vi "Simulated LIDAR (Faster).vi"(8 "error in (no error)":errorcluster, 9 "End Point (120°)":dbl=120.0, 10 "Start Point (-120°)":dbl=-120.0) -> (0 "error out":errorcluster, 1 "Direction":dbl[](array[numeric]), 2 "Magnitude":dbl[](array[numeric]))   [LabVIEW 2011]
doc: "This VI takes three parameters (start point, end point, cluster count) and returns two arrays which describe the magnitude and angle at which the data was acquired. \n\nThe reference for the angles (in the Direction array) is the center of the device which is 0° with positive angles to the left of center and negative angles to the right.\n\nThe URG-04LX can take measurements in the range of -120° to 120° and has an \"operating range\" of -135° to 135°. \n\nCluster Count refers to the number of measurements which are clustered together. \n<b>Ex:</b>If the cluster count is 3 then the smallest of three measurements is returned.\n\nThe Magnitude array is associated with the Direction array. \n<b>Ex:</b> If the information for the first measurement is desired, then the 0th index of each array is accessed and returns the magnitude and direction of the first measurement.\n\nIf checksums are being used and the checksum fails, the data returned in the magnitude array will default to -1."
uses:
  2D Point.ctl
  <vilib>/Analysis/coordinate.llb/Wrap Angle (scalar).vi
  <vilib>/Analysis/coordinate.llb/2D Cartesian Coordinate Rotation (Scalar).vi
  <vilib>/Utility/AngleManip/Radians to Degrees (Scalar DBL).vi
  <vilib>/Utility/AngleManip/Degrees to Radians (Scalar DBL).vi
  <vilib>/Analysis/NI_AALPro.lvlib
  <vilib>/Analysis/NI_AALBase.lvlib
  <vilib>/Utility/AngleManip/NI_AngleManipulation.lvlib
  <vilib>/Analysis/NI_AAL_Angle.lvlib
panel:
  in  "Add noise?":bool=TRUE
  in  "noise (standard deviation)":dbl=30.0
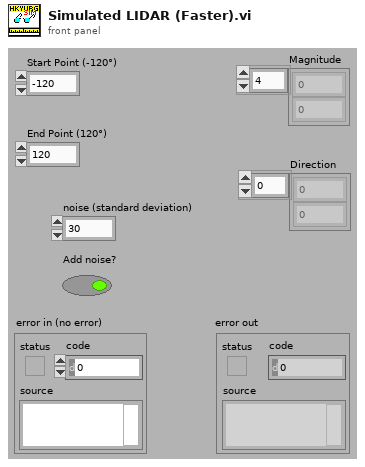
[diagram p1: front panel]
types:
  T1 = typedef "2D Point.ctl" = cluster{"X":dbl, "Y":dbl}
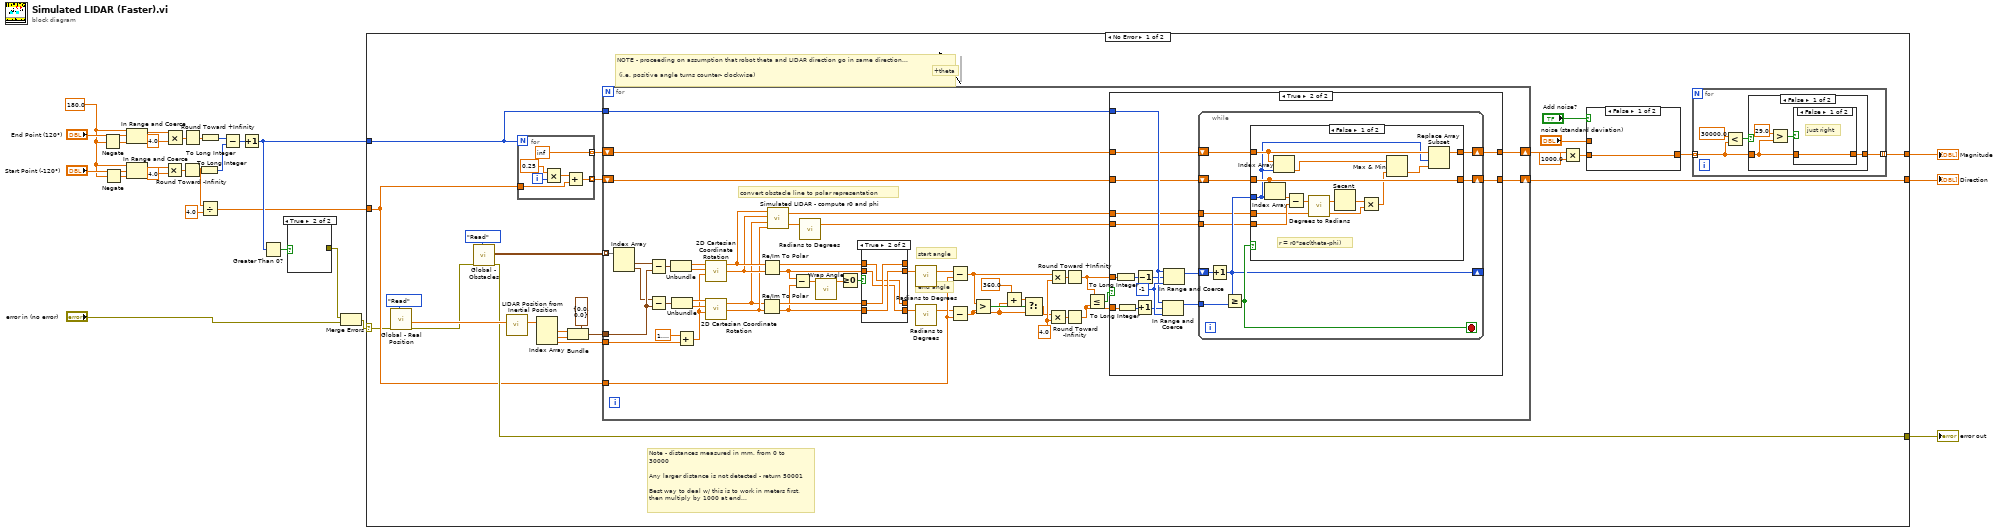
[diagram p0: block diagram]
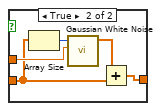
[diagram p2: hidden frame]
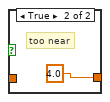
[diagram p3: hidden frame]
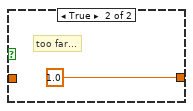
[diagram p4: hidden frame]
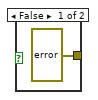
[diagram p9: hidden frame]
diagram:
  w20 = 180.0 ("upper limit")
  n1 = Negate(x=w20) -> (-x=w22:dbl)
  n2 = Negate(x=w20) -> (-x=w23:dbl)
  n3 = In Range and Coerce(upper limit=w20, x="End Point (120°)", lower limit=w22) -> (coerced(x)=w18:dbl)  [unwired: 1 out]
  n4 = In Range and Coerce(upper limit=w20, x="Start Point (-120°)", lower limit=w23) -> (coerced(x)=w19:dbl)  [unwired: 1 out]
  n5 = Multiply(x=w19, y=4.0) -> (x*y=w6:dbl)
  n6 = Multiply(x=w18, y=4.0) -> (x*y=w25:dbl)
  n7 = Round Toward -Infinity(1:w6) -> (0:w4:dbl)
  n8 = Round Toward +Infinity(x=w25) -> (ceil(x): smallest int >= x=w17:dbl)
  n9 = To Long Integer(number=w4) -> (32bit integer=w16:i32)
  n10 = To Long Integer(number=w17) -> (32bit integer=w15:i32)
  n11 = Divide(x=w4, y=4.0) -> (x/y=w3:dbl)
  n12 = Subtract(x=w15, y=w16) -> (x-y=w14:i32)
  n13 = Increment(x=w14) -> (x+1=w11:i32)
  n14 = Greater Than 0?(x=w11) -> (x > 0?=w9:bool)
  n15 = case shown="True" w9 {
    tunnel: [errorcluster {"status"=TRUE, "code"=1, "source"="Simulated LIDAR: Check Start and End Points"} ("t") _] -> w8
    frame False {
    }
    frame True {
    }
  }
  n16 = Merge Errors(w8, "error in (no error)") -> (w7:errorcluster)
  n17 = case shown="No Error" w7 {
    selector: w7 -> [w28 _]
    tunnel: [w44 _] -> w12
    tunnel: w11 -> [w37 _]
    tunnel: w3 -> [w38 _]
    tunnel: [w36 _] -> w2
    tunnel: [w34 _] -> w1
    frame No Error {
      # "NOTE - proceeding on assumption that robot theta and LIDAR direction go in same direction...\n\n (i.e. positive angle turns counter- clockwise)"
      # "+theta"
      # "Note - distances measured in mm, from 0 to 30000\n\nAny larger distance is not detected - return 50001\n\nBest way to deal w/ this is to work in meters first, then multiply by 1000 at end..."
      n18 = call "Global - Real Position.vi"("mode"=enum16{"Initialize", "Read", "Write"}."Read" ("Mode"), "error in (no error)"=w28) -> ("error out"=w46:errorcluster, "real x, y, theta out"=w48:dbl[])  [unwired: 7 in, 1 out]
      n19 = call "Global - Obstacles.vi"("mode"=enum16{"Initialize", "Read", "Write"}."Read" ("Mode"), "error in (no error)"=w46) -> ("error out"=w44:errorcluster, "obstacles out"=w43:cluster{dbl, dbl}[][])  [unwired: 7 in, 1 out]
      n20 = call "LIDAR Position from Inertial Position.vi"("CM X, Y, Theta"=w48) -> ("LIDAR X, Y, Theta"=w47:dbl[])  [unwired: 1 in, 9 out]
      n21 = for {
        N: w37 -> [_]
        tunnel: [inf] -> w39 mode=indexing
        tunnel: w38 -> [w71]
        tunnel: [w70] -> w40 mode=indexing
        i -> [w74]
        n22 = Multiply(x=0.25, y=w74) -> (x*y=w73:dbl)
        n23 = Add(x=w73, y=w71) -> (x+y=w70:dbl)
      }
      n24 = Index Array(array=w47) -> (element #1=w51:dbl, element #2=w50:dbl, element #3=w41:dbl)  [unwired: 3 in]
      n25 = Bundle(cluster=T1 {"X"=0.0, "Y"=0.0} ("2D Point"), "X"=w51, "Y"=w50) -> (w42:T1)
      n26 = for {
        tunnel: w43 -> [w124] mode=indexing
        tunnel: w42 -> [w123]
        tunnel: w41 -> [w86]
        shift-right: [w88] -> w36
        shift-left: w40 -> [w89]
        shift-right: [w90] -> w33
        shift-left: w39 -> [w91]
        tunnel: w38 -> [w105]
        tunnel: w37 -> [w101]
        w104 = 4.0 ("y")
        # "convert obstacle line to polar representation"
        # "end angle"
        # "start angle"
        n27 = Index Array(array=w124) -> (element #1=w122:cluster{dbl, dbl}, element #2=w121:cluster{dbl, dbl})  [unwired: 2 in]
        n28 = Subtract(x=w122, y=w123) -> (x-y=w120:T1)
        n29 = Subtract(x=w121, y=w123) -> (x-y=w119:T1)
        n30 = Unbundle(w120) -> ("X"=w118:dbl, "Y"=w117:dbl)
        n31 = Unbundle(w119) -> ("X"=w116:dbl, "Y"=w115:dbl)
        n32 = Add(x=1.5707963267948966, y=w86) -> (x+y=w85:dbl)
        n33 = call-poly <vilib>:"2D Cartesian Coordinate Rotation.vi"("theta"=w85, "y"=w117, "x"=w118) -> ("y out"=w108:dbl, "x out"=w109:dbl)  [unwired: 6 in, 1 out]
        n34 = call-poly <vilib>:"2D Cartesian Coordinate Rotation.vi"("theta"=w85, "y"=w115, "x"=w116) -> ("y out"=w107:dbl, "x out"=w106:dbl)  [unwired: 6 in, 1 out]
        n35 = Re/Im To Polar(2:w107, 3:w106) -> (0:w110:dbl, 1:w111:dbl)
        n36 = Re/Im To Polar(2:w108, 3:w109) -> (0:w112:dbl, 1:w113:dbl)
        n37 = call "Simulated LIDAR - compute r0 and phi.vi"("y2"=w107, "x2"=w106, "y1"=w108, "x1"=w109) -> ("phi"=w83:dbl, "r0"=w87:dbl)
        n38 = Subtract(x=w112, y=w110) -> (x-y=w77:dbl)
        n39 = call-poly <vilib>:"Radians to Degrees.vi"("angle (rad)"=w83) -> ("angle (deg)"=w82:dbl)  [unwired: 2 in]
        n40 = call-poly <vilib>:"Wrap Angle.vi"("angle in"=w77) -> ("angle out"=w76:dbl)  [unwired: 9 in, 1 out]
        n41 = Greater Or Equal To 0?(x=w76) -> (x >= 0?=w114:bool)
        n42 = case shown="True" w114 {
          tunnel: w113 -> [w171 w173]
          tunnel: w112 -> [w170 w172]
          tunnel: w111 -> [w169 w175]
          tunnel: w110 -> [w168 w174]
          tunnel: [w171 w175] -> _
          tunnel: [w170 w174] -> w79
          tunnel: [w169 w173] -> _
          tunnel: [w168 w172] -> w81
          frame False {
          }
          frame True {
          }
        }
        n43 = call-poly <vilib>:"Radians to Degrees.vi"("angle (rad)"=w79) -> ("angle (deg)"=w78:dbl)  [unwired: 2 in]
        n44 = call-poly <vilib>:"Radians to Degrees.vi"("angle (rad)"=w81) -> ("angle (deg)"=w80:dbl)  [unwired: 2 in]
        n45 = Subtract(x=w78, y=w105) -> (x-y=w100:dbl)
        n46 = Subtract(x=w80, y=w105) -> (x-y=w96:dbl)
        n47 = Greater?(x=w100, y=w96) -> (0:w97:bool)
        n48 = Add(x=360.0, y=w96) -> (x+y=w99:dbl)
        n49 = Select(t=w99, s=w97, f=w96) -> (s? t:f=w95:dbl)
        n50 = Multiply(x=w95, y=w104) -> (x*y=w102:dbl)
        n51 = Multiply(x=w100, y=w104) -> (x*y=w103:dbl)
        n52 = Round Toward +Infinity(x=w103) -> (ceil(x): smallest int >= x=w94:dbl)
        n53 = Round Toward -Infinity(1:w102) -> (0:w93:dbl)
        n54 = Less Or Equal?(x=w94, y=w93) -> (x <= y?=w92:bool)
        n55 = case shown="True" w92 {
          tunnel: w101 -> [_ w139]
          tunnel: w94 -> [_ w138]
          tunnel: w93 -> [_ w137]
          tunnel: w91 -> [w126 w132]
          tunnel: [w126 w131] -> w90
          tunnel: w89 -> [w125 w130]
          tunnel: [w125 w129] -> w88
          tunnel: w82 -> [_ w128]
          tunnel: w87 -> [_ w127]
          frame False {
          }
          frame True {
            w140 = -1 ("lower limit")
            n56 = To Long Integer(number=w138) -> (32bit integer=w142:i32)
            n57 = To Long Integer(number=w137) -> (32bit integer=w141:i32)
            n58 = Increment(x=w141) -> (x+1=w135:i32)
            n59 = Decrement(x=w142) -> (x-1=w136:i32)
            n60 = In Range and Coerce(upper limit=w139, x=w135, lower limit=w140) -> (coerced(x)=w133:i32)  [unwired: 1 out]
            n61 = In Range and Coerce(upper limit=w139, x=w136, lower limit=w140) -> (coerced(x)=w134:i32)  [unwired: 1 out]
            n62 = while {
              shift-right: [w148] -> _
              shift-left: w134 -> [w149]
              tunnel: w133 -> [w152]
              shift-right: [w145] -> w131
              shift-left: w132 -> [w144]
              shift-right: [w143] -> w129
              shift-left: w130 -> [w150]
              tunnel: w128 -> [w147]
              tunnel: w127 -> [w146]
              stop <- w151 stop-if-true
              n63 = Increment(x=w149) -> (x+1=w148:i32)
              n64 = Greater Or Equal?(x=w148, y=w152) -> (x >= y?=w151:bool)
              n65 = case shown="False" w151 {
                tunnel: w150 -> [w160 w166]
                tunnel: w148 -> [w156 _]
                tunnel: w147 -> [w164 _]
                tunnel: w146 -> [w162 _]
                tunnel: [w161 w167] -> w145
                tunnel: w144 -> [w159 w167]
                tunnel: [w160 w166] -> w143
                frame False {
                  # "r = r0*sec(theta-phi)"
                  n66 = Index Array(array=w160, index=w156) -> (element=w165:dbl)
                  n67 = Index Array(array=w159, index=w156) -> (element=w158:dbl)
                  n68 = Subtract(x=w165, y=w164) -> (x-y=w154:dbl)
                  n69 = call-poly <vilib>:"Degrees to Radians.vi"("angle (deg)"=w154) -> ("angle (rad)"=w153:dbl)  [unwired: 2 in]
                  n70 = Secant(1:w153) -> (0:w163:dbl)
                  n71 = Multiply(x=w163, y=w162) -> (x*y=w157:dbl)
                  n72 = Max & Min(x=w158, y=w157) -> (min(x,y)=w155:dbl)  [unwired: 1 out]
                  n73 = Replace Array Subset(array=w159, new element=w155, index=w156) -> (w161:dbl[])
                }
                frame True {
                }
              }
            }
          }
        }
      }
      n74 = Multiply(x=w33, y=1000.0) -> (x*y=w31:dbl[])
      n75 = case shown="False" "Add noise?" {
        tunnel: "noise (standard deviation)" -> [_ w57]
        tunnel: w31 -> [w53 w55]
        tunnel: [w53 w54] -> w29
        frame False {
        }
        frame True {
          n76 = Array Size(array=w55) -> (size(s)=w58:i32)
          n77 = call <vilib>:"Gaussian White Noise.vi"("standard deviation"=w57, "samples"=w58) -> ("Gaussian noise pattern"=w56:dbl[])  [unwired: 8 in, 1 out]
          n78 = Add(x=w56, y=w55) -> (x+y=w54:dbl[])
        }
      }
      n79 = for {
        tunnel: w29 -> [w60] mode=indexing
        tunnel: [w59] -> w34 mode=indexing
        n80 = Less?(x=30000.0 ("y"), y=w60) -> (x < y?=w61:bool)
        n81 = case shown="False" w61 {
          tunnel: w60 -> [w64 _]
          tunnel: [w63 1.0 ("f")] -> w59
          frame False {
            n82 = Greater?(x=29.0 ("y"), y=w64) -> (0:w65:bool)
            n83 = case shown="False" w65 {
              tunnel: w64 -> [w67 _]
              tunnel: [w67 4.0 ("y")] -> w63
              frame False {
                # "just right"
              }
              frame True {
                # "too near"
              }
            }
          }
          frame True {
            # "too far..."
          }
        }
      }
    }
    frame Error {
    }
  }
  "Magnitude" <- w1
  "Direction" <- w2
  "error out" <- w12
